vi "GV DOdelay_tick.vi"() -> ()   [LabVIEW 2017]
panel:
  in  "DOdelay_tick":u32
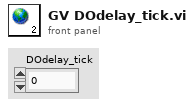
[diagram p1: front panel]
diagram:
